vi "_rep_cap_variant_to_cmd_value_string.vi"(5 "RepCap value in":variant, 6 "Error creation enabled (T)":bool=TRUE, 7 "RepCapName in":string, 8 "error in":errorcluster caption="error in (no error)", 9 "RepCap Type in":T1, 11 "RepCapName ID in":string) -> (0 "error out":errorcluster, 2 "Error occured":bool=TRUE, 3 "CmdValue out":string)   [LabVIEW 2022 SP3, in "hmp4000_rsidr_core.lvlib"]
uses:
  hmp4000_rsidr_core.lvlib
  _type_RepCap_Type.ctl
  type_Error_Codes.ctl
  Trim Whitespace One-Sided.vi
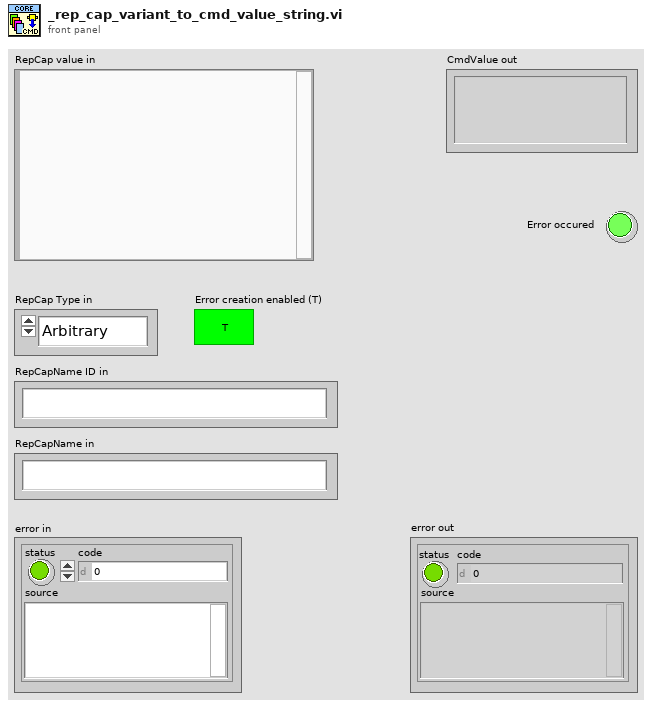
[diagram p1: front panel]
types:
  T1 = typedef "hmp4000_rsidr_core.lvlib/_type_RepCap_Type.ctl" = enum16{"Arbitrary", "SequentialNull", "Sequential"}
  T2 = typedef "hmp4000_rsidr_core.lvlib/type_Error_Codes.ctl" = enum16{"No_error", "VISA_err_ResourceNotFound", "VISA_err_Timeout", "VISA_warn_MoreDataAvailable", "RS_err_MissingCallback", "RS_err_InvalidAttribute", "RS_err_InvalidValue", "RS_err_UnknownResource", "RS_err_AlreadyInitialized", "RS_err_InstrumentStatus", "RS_err_BadRepCapName", "RS_err_TypesMismatch", "RS_err_ValueNotSupported", "RS_err_InvalidRngTable", "RS_err_IDqueryFail", "RS_err_UnexpResponse", "VISA_warn_ConfigNotLoaded", "RS_err_AttributeNotReadable", "RS_err_AttributeNotWritable", "RS_err_InstrumentType", "RS_err_InstrumentOption", "VISA_err_InvalidSize", "RS_err_ReliabilityIndicator", "VISA_warn_UnknownStatus", "VISA_warn_TermCharRead", "VISA_err_IO_error", "RS_err_FunctionNotSupported", "VISA_warn_QueueEmpty"}
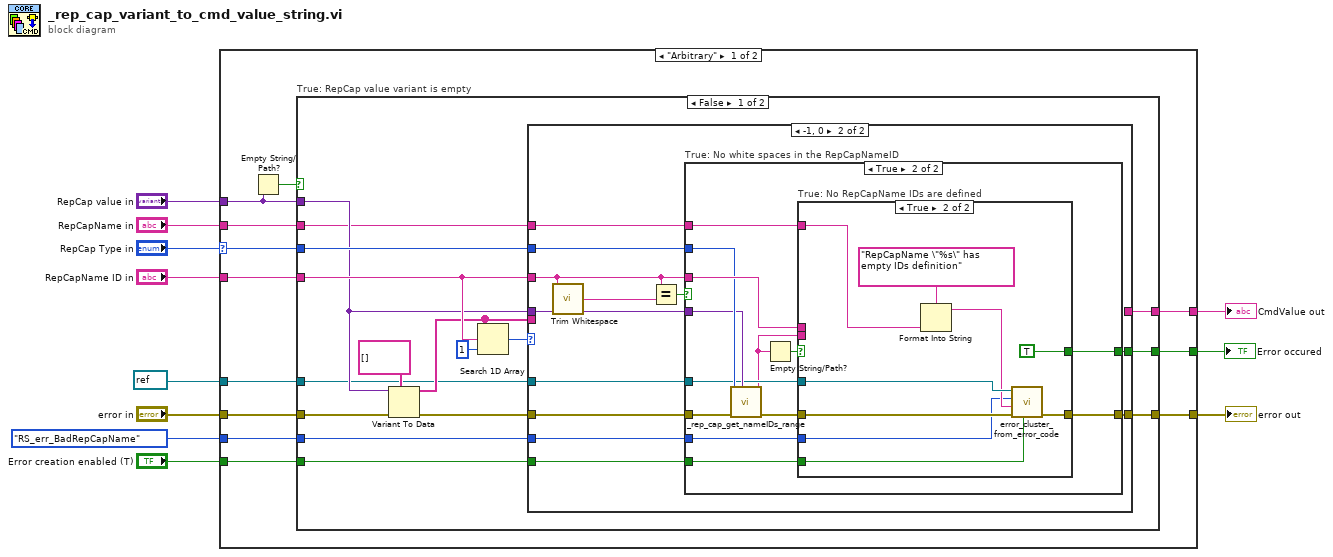
[diagram p0: block diagram]
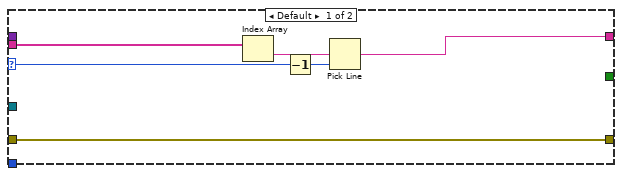
[diagram p2: hidden frame]
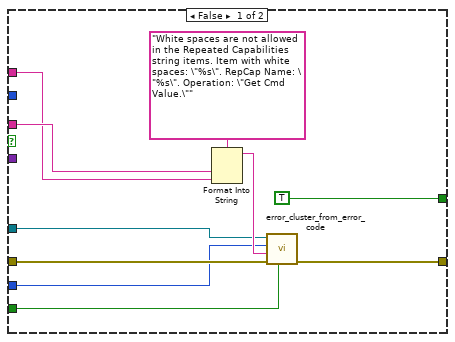
[diagram p3: hidden frame]
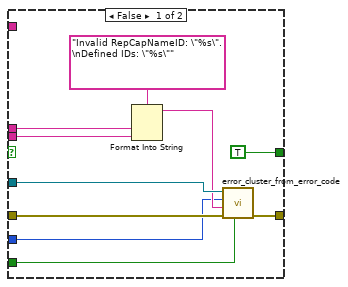
[diagram p4: hidden frame]
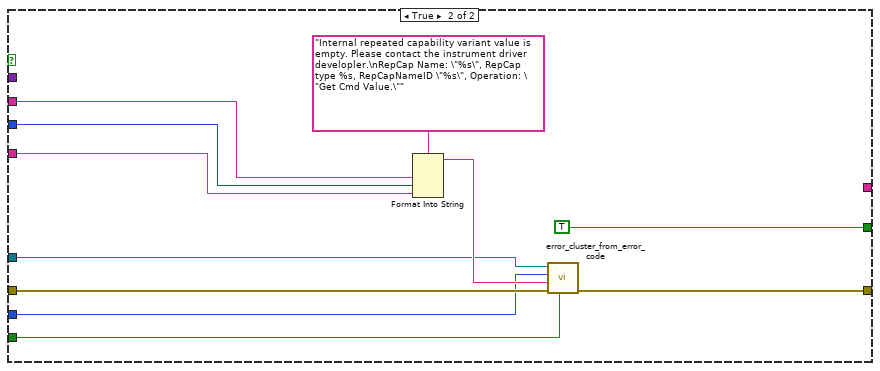
[diagram p5: hidden frame]
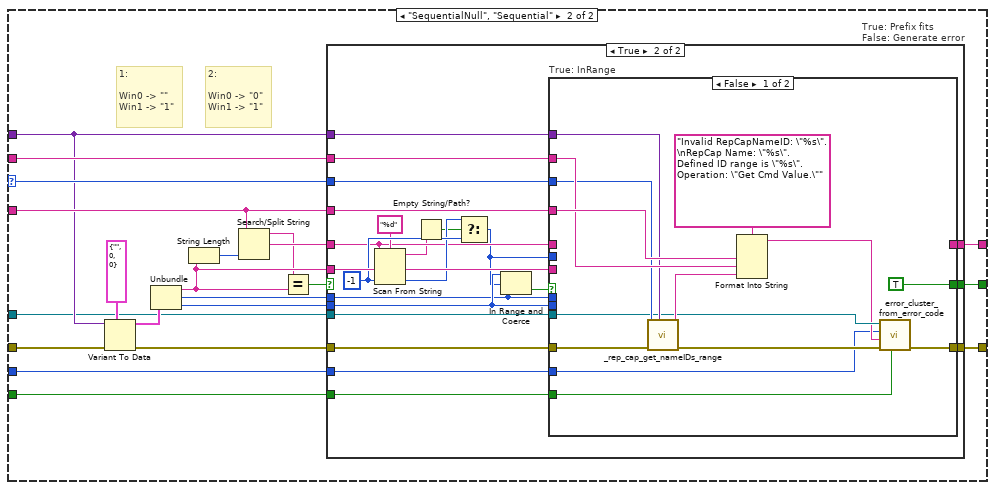
[diagram p6: hidden frame]
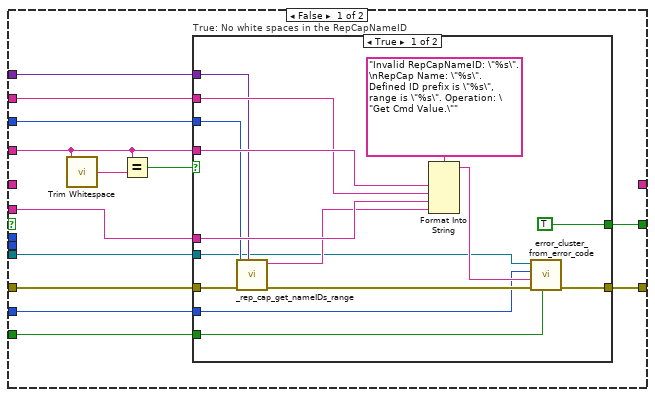
[diagram p7: hidden frame]
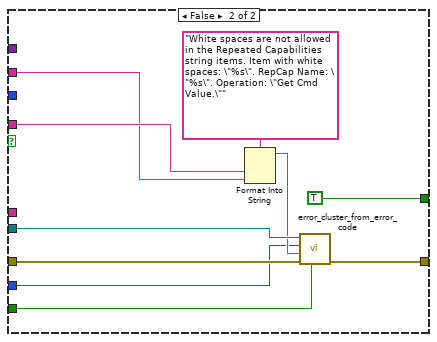
[diagram p8: hidden frame]
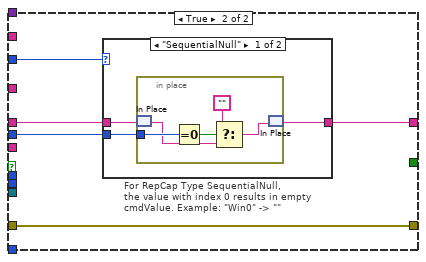
[diagram p9: hidden frame]
diagram:
  n1 = case shown="\"Arbitrary\"" "RepCap Type in" {
    selector: "RepCap Type in" -> [w19 w123]
    tunnel: "RepCapName ID in" -> [w20 w128]
    tunnel: [w21 w122] -> w4
    tunnel: "RepCap value in" -> [w17 w115]
    tunnel: "error in" -> [w23 w131]
    tunnel: [w22 w124] -> w5
    tunnel: "RepCapName in" -> [w18 w116]
    tunnel: refnum<visa-resource-name> refnum ("VISA resource name") -> [w15 w114]
    tunnel: "Error creation enabled (T)" -> [w14 w113]
    tunnel: [w13 w112] -> w2
    tunnel: type_Error_Codes."RS_err_BadRepCapName" ("ErrorCodes") -> [w12 w111]
    frame "Arbitrary" {
      n2 = Empty String/Path?(string/path=w17) -> (empty?=w16:bool)
      n3 = case "True: RepCap value variant is empty" shown="False" w16 {
        tunnel: w23 -> [w39 w110]
        tunnel: [w35 w109] -> w22
        tunnel: [w33 _] -> w21
        tunnel: w20 -> [w32 w105]
        tunnel: w19 -> [w30 w106]
        tunnel: w17 -> [w29 _]
        tunnel: w18 -> [w28 w107]
        tunnel: w15 -> [w24 w103]
        tunnel: w12 -> [w27 w102]
        tunnel: w14 -> [w25 w101]
        tunnel: [w26 TRUE] -> w13
        frame False {
          n4 = Variant To Data(error in=w39, type=string[] [], Variant=w29) -> (data=w31:string[], error out=w36:errorcluster)
          n5 = Search 1D Array(1D array=w31, element=w32, start index (0)=1) -> (index of element=w34:i32)
          n6 = case shown="-1, 0" w34 {
            selector: w34 -> [w44 _]
            tunnel: w36 -> [w45 w56]
            tunnel: [w45 w57] -> w35
            tunnel: [w40 _] -> w33
            tunnel: w31 -> [w42 _]
            tunnel: w32 -> [_ w52]
            tunnel: w30 -> [_ w55]
            tunnel: w29 -> [_ w54]
            tunnel: w28 -> [_ w50]
            tunnel: w24 -> [_ w49]
            tunnel: w27 -> [_ w48]
            tunnel: [_ w47] -> w26
            tunnel: w25 -> [_ w46]
            frame Default {
              n7 = Index Array(array=w42) -> (element=w41:string)  [unwired: 1 in]
              n8 = Decrement(x=w44) -> (x-1=w43:i32)
              n9 = Pick Line(multi-line string=w41, line index=w43) -> (output string=w40:string)  [unwired: 1 in]
            }
            frame -1, 0 {
              n10 = call "Trim Whitespace.vi"("string"=w52) -> ("trimmed string"=w53:string)  [unwired: 1 in]
              n11 = Equal?(x=w52, y=w53) -> (x = y?=w51:bool)
              n12 = case "True: No white spaces in the RepCapNameID" shown="True" w51 {
                tunnel: [w65 w80] -> w57
                tunnel: w52 -> [w64 w79]
                tunnel: w56 -> [w66 w78]
                tunnel: w55 -> [_ w76]
                tunnel: w54 -> [_ w75]
                tunnel: w50 -> [w63 w71]
                tunnel: w49 -> [w61 w74]
                tunnel: w48 -> [w60 w70]
                tunnel: [TRUE w69] -> w47
                tunnel: w46 -> [w59 w68]
                frame False {
                  n13 = Format Into String(format string="White spaces are not allowed in the Repeated Capabilities string items. Item with white spaces: \"%s\". RepCap Name: \"%s\". Operation: \"Get Cmd Value.\"" ("error message (\"\")"), w64, w63) -> (resulting string=w62:string)  [unwired: 2 in, 1 out]
                  n14 = call "error_cluster_from_error_code.vi"("Error Creation Enabled (True)"=w59, "error in"=w66, "Error Message (\"\")"=w62, "Error Enum in"=w60, "VISA resource name"=w61) -> ("error out"=w65:errorcluster)  [unwired: 5 in, 1 out]
                }
                frame True {
                  n15 = call "_rep_cap_get_nameIDs_range.vi"("RepCap value in"=w75, "error in"=w78, "RepCap Type in"=w76) -> ("error out"=w77:errorcluster, "ID range out"=w72:string)  [unwired: 6 in, 1 out]
                  n16 = Empty String/Path?(string/path=w72) -> (empty?=w73:bool)
                  n17 = case "True: No RepCapName IDs are defined" shown="True" w73 {
                    tunnel: [w89 w98] -> w80
                    tunnel: w79 -> [w88 _]
                    tunnel: w77 -> [w87 w97]
                    tunnel: w72 -> [w86 _]
                    tunnel: w74 -> [w85 w96]
                    tunnel: w71 -> [_ w94]
                    tunnel: w70 -> [w83 w93]
                    tunnel: [TRUE TRUE] -> w69
                    tunnel: w68 -> [w81 w92]
                    frame False {
                      n18 = Format Into String(format string="Invalid RepCapNameID: \"%s\".\nDefined IDs: \"%s\"" ("error message (\"\")"), w88, w86) -> (resulting string=w84:string)  [unwired: 2 in, 1 out]
                      n19 = call "error_cluster_from_error_code.vi"("Error Creation Enabled (True)"=w81, "error in"=w87, "Error Message (\"\")"=w84, "Error Enum in"=w83, "VISA resource name"=w85) -> ("error out"=w89:errorcluster)  [unwired: 5 in, 1 out]
                    }
                    frame True {
                      n20 = Format Into String(format string="RepCapName \"%s\" has empty IDs definition" ("error message (\"\")"), w94) -> (resulting string=w95:string)  [unwired: 2 in, 1 out]
                      n21 = call "error_cluster_from_error_code.vi"("Error Creation Enabled (True)"=w92, "error in"=w97, "Error Message (\"\")"=w95, "Error Enum in"=w93, "VISA resource name"=w96) -> ("error out"=w98:errorcluster)  [unwired: 5 in, 1 out]
                    }
                  }
                }
              }
            }
          }
        }
        frame True {
          n22 = Format Into String(format string="Internal repeated capability variant value is empty. Please contact the instrument driver developler.\nRepCap Name: \"%s\", RepCap type %s, RepCapNameID \"%s\", Operation: \"Get Cmd Value.\"" ("error message (\"\")"), w107, w106, w105) -> (resulting string=w104:string)  [unwired: 2 in, 1 out]
          n23 = call "error_cluster_from_error_code.vi"("Error Creation Enabled (True)"=w101, "error in"=w110, "Error Message (\"\")"=w104, "Error Enum in"=w102, "VISA resource name"=w103) -> ("error out"=w109:errorcluster)  [unwired: 5 in, 1 out]
        }
      }
    }
    frame "SequentialNull", "Sequential" {
      # "1:\n\nWin0 -> \"\"\nWin1 -> \"1\""
      # "2:\n\nWin0 -> \"0\"\nWin1 -> \"1\""
      n24 = Variant To Data(error in=w131, type=cluster{string, i32, i32} {"", 0, 0} ("output cluster"), Variant=w115) -> (data=w117:cluster{string, i32, i32}, error out=w130:errorcluster)
      n25 = Unbundle(w117) -> (w121:string, w119:i32, w125:i32)
      n26 = String Length(string=w121) -> (length=w129:i32)
      n27 = Search/Split String(string=w128, offset (0)=w129) -> (substring before match=w120:string, match + rest of string=w126:string)  [unwired: 1 in, 1 out]
      n28 = Equal?(x=w120, y=w121) -> (x = y?=w127:bool)
      n29 = case "True: Prefix fits\nFalse: Generate error" shown="True" w127 {
        tunnel: w130 -> [w141 w191]
        tunnel: w128 -> [w132 w188]
        tunnel: w126 -> [_ w172]
        tunnel: w119 -> [_ w186]
        tunnel: w125 -> [_ w187]
        tunnel: [w144 w190] -> w124
        tunnel: w123 -> [w140 w185]
        tunnel: [_ w184] -> w122
        tunnel: w121 -> [w143 w183]
        tunnel: w116 -> [w142 w182]
        tunnel: w115 -> [w139 w181]
        tunnel: w114 -> [w136 w180]
        tunnel: w111 -> [w135 w179]
        tunnel: w113 -> [w134 w178]
        tunnel: [w133 w177] -> w112
        frame False {
          n30 = call "Trim Whitespace.vi"("string"=w132) -> ("trimmed string"=w138:string)  [unwired: 1 in]
          n31 = Equal?(x=w132, y=w138) -> (x = y?=w137:bool)
          n32 = case "True: No white spaces in the RepCapNameID" shown="True" w137 {
            tunnel: [w158 w168] -> w144
            tunnel: w132 -> [w157 w167]
            tunnel: w143 -> [w156 _]
            tunnel: w142 -> [w155 w166]
            tunnel: w141 -> [w154 w165]
            tunnel: w140 -> [w152 _]
            tunnel: w139 -> [w151 _]
            tunnel: w136 -> [w145 w164]
            tunnel: w135 -> [w148 w162]
            tunnel: w134 -> [w147 w161]
            tunnel: [TRUE TRUE] -> w133
            frame True {
              n33 = call "_rep_cap_get_nameIDs_range.vi"("RepCap value in"=w151, "error in"=w154, "RepCap Type in"=w152) -> ("error out"=w153:errorcluster, "ID range out"=w150:string)  [unwired: 6 in, 1 out]
              n34 = Format Into String(format string="Invalid RepCapNameID: \"%s\".\nRepCap Name: \"%s\". Defined ID prefix is \"%s\", range is \"%s\". Operation: \"Get Cmd Value.\"" ("error message (\"\")"), w157, w155, w156, w150) -> (resulting string=w149:string)  [unwired: 2 in, 1 out]
              n35 = call "error_cluster_from_error_code.vi"("Error Creation Enabled (True)"=w147, "error in"=w153, "Error Message (\"\")"=w149, "Error Enum in"=w148, "VISA resource name"=w145) -> ("error out"=w158:errorcluster)  [unwired: 5 in, 1 out]
            }
            frame False {
              n36 = Format Into String(format string="White spaces are not allowed in the Repeated Capabilities string items. Item with white spaces: \"%s\". RepCap Name: \"%s\". Operation: \"Get Cmd Value.\"" ("error message (\"\")"), w167, w166) -> (resulting string=w163:string)  [unwired: 2 in, 1 out]
              n37 = call "error_cluster_from_error_code.vi"("Error Creation Enabled (True)"=w161, "error in"=w165, "Error Message (\"\")"=w163, "Error Enum in"=w162, "VISA resource name"=w164) -> ("error out"=w168:errorcluster)  [unwired: 5 in, 1 out]
            }
          }
        }
        frame True {
          w176 = -1 ("default value 1")
          n38 = Scan From String(format string="%d", input string=w172, default 1=w176) -> (remaining string=w170:string, output 1=w175:i32)  [unwired: 2 in, 2 out]
          n39 = Empty String/Path?(string/path=w170) -> (empty?=w174:bool)
          n40 = Select(t=w175, s=w174, f=w176) -> (s? t:f=w171:i32)
          n41 = In Range and Coerce(upper limit=w187, x=w171, lower limit=w186) -> (In Range?=w189:bool)  [unwired: 1 out]
          n42 = case "True: InRange" shown="False" w189 {
            tunnel: w191 -> [w201 w206]
            tunnel: [w204 w206] -> w190
            tunnel: w188 -> [w203 _]
            tunnel: w172 -> [_ w209]
            tunnel: w186 -> [_ _]
            tunnel: w187 -> [_ _]
            tunnel: w185 -> [w199 w210]
            tunnel: [_ w208] -> w184
            tunnel: w171 -> [_ w207]
            tunnel: w183 -> [_ _]
            tunnel: w182 -> [w202 _]
            tunnel: w181 -> [w198 _]
            tunnel: w180 -> [w196 _]
            tunnel: w179 -> [w194 _]
            tunnel: w178 -> [w193 _]
            tunnel: [TRUE _] -> w177
            frame False {
              n43 = call "_rep_cap_get_nameIDs_range.vi"("RepCap value in"=w198, "error in"=w201, "RepCap Type in"=w199) -> ("error out"=w200:errorcluster, "ID range out"=w197:string)  [unwired: 6 in, 1 out]
              n44 = Format Into String(format string="Invalid RepCapNameID: \"%s\".\nRepCap Name: \"%s\". Defined ID range is \"%s\". Operation: \"Get Cmd Value.\"" ("error message (\"\")"), w203, w202, w197) -> (resulting string=w195:string)  [unwired: 2 in, 1 out]
              n45 = call "error_cluster_from_error_code.vi"("Error Creation Enabled (True)"=w193, "error in"=w200, "Error Message (\"\")"=w195, "Error Enum in"=w194, "VISA resource name"=w196) -> ("error out"=w204:errorcluster)  [unwired: 5 in, 1 out]
            }
            frame True {
              n46 = case "For RepCap Type SequentialNull,\nthe value with index 0 results in empty\ncmdValue. Example: \"Win0\" -> \"\"" shown="\"SequentialNull\"" w210 {
                tunnel: w209 -> [w212 w219]
                tunnel: [w211 w219] -> w208
                tunnel: w207 -> [w213 _]
                frame "SequentialNull" {
                  n47 = in-place "In Place Element Structure" {
                    in-place-border: w213 -> [w218]
                    n48 = in-place-match #1 ("In Place In / Out Element")(w212) -> (w215:string)
                    n49 = Equal To 0?(x=w218) -> (x = 0?=w217:bool)
                    n50 = Select(t="" ("Empty String Constant"), s=w217, f=w215) -> (s? t:f=w214:string)
                    n51 = in-place-match #1 ("In Place In / Out Element")(w214) -> (w211:string)
                  }
                }
                frame "Arbitrary", "Sequential" {
                }
              }
            }
          }
        }
      }
    }
  }
  "CmdValue out" <- w4
  "error out" <- w5
  "Error occured" <- w2
